vi "Tom Comparison.vi"(8 "Settings":T2={"Name of test"="hammer test--hammer test 03", "Date"=timestamp(3831903982 s since 1904-01-01), "Location"="Home", "Template"="ScratchPad", "Soundcard"="1-2 (QUAD-CAPTURE)", "resolution"=32, "Sampling rate"=48000, "Ch1 Gain "=0.0, "Ch2 Gain"=0.0, "Sample time (s)"=0.3, "Pre-trigger (s)"=0.001, "Hammer Threshold"=0.01, "Positions"=2, "Taps/Position"=5, "Set Names"="H", "Freq resolution"=1.0, "Hammer cutoff"=0.0016020942408376962, "Mic cutoff"=0.06, "Double bounce "=0.01, "Hammer Cal"=1.0, "dB Offset"=0.0, "Accel Cal"=1.0, "Vibrometer Cal"=40.0, "Mic Cal"=66.0, "Output"=0, "Voltage Cal"=1.0, "Vibrometer Port"="ASRL27::INSTR", "Range"=20, "High Pass"=0, "Bandwidth"=25, "X Range"=[{"Minimum"=200.0, "Maximum"=20000.0, "Increment"=10.0, "Minor Increment"=100.0, "Start"=1000.0}, {"Minimum"=0.0, "Maximum"=0.002, "Increment"=0.0005, "Minor Increment"=0.0001, "Start"=0.0}, {"Minimum"=-0.02, "Maximum"=0.3, "Increment"=0.1, "Minor Increment"=0.01, "Start"=0.0}, {"Minimum"=150.0, "Maximum"=10000.0, "Increment"=10.0, "Minor Increment"=100.0, "Start"=1000.0}], "Y Range"=[{"Minimum"=-25.0, "Maximum"=0.0, "Increment"=5.0, "Minor Increment"=1.0, "Start"=-25.0}, {"Minimum"=-0.01, "Maximum"=0.1, "Increment"=0.025, "Minor Increment"=0.005, "Start"=0.0}, {"Minimum"=-1.0, "Maximum"=1.0, "Increment"=0.5, "Minor Increment"=0.1, "Start"=-1.0}, {"Minimum"=0.0, "Maximum"=40.0, "Increment"=2.0, "Minor Increment"=0.5, "Start"=0.0}], "dB Spread"=40.0, "Trigger"=0, "Ch_1"=2, "Ch_2"=1, "flip?"=FALSE, "60Hz"=FALSE, "Time offset"=0.0, "Piezo Cal"=1.0, "Default Notes"="location (e.g., JC workshop, Oberlin acoustics, etc.)\nname of experiment (if applicable) \nnames of researchers\n\nInstrument Information:\ninstrument (e.g., violin, viola, cello, guitar, mandolin, etc.) \nmodel (e.g., Titian Strad, Guadagnini, personal, etc.) \nmaker name\nmaker ID (e.g., serial number)\nyear built (4 digits)\ncountry of origin \nsession (e.g. Oberlin 2017, VSA 2008) \nmaking school (e.g. Old Italian) \n\nMeasurement Information:\ntype (Radiation, admittance, modal analysis, taptones, etc.) \nprotocol (HV24, etc.)\n"} {"Ch_2" min=1 step=1; "Ch_1" min=1 max=100 step=1; "Trigger" items=["Hammer (force)", "Self-tap", "Spacebar"]; "Bandwidth" items=["1 kHz"=1, "5 kHz"=5, "10 kHz"=10, "25 kHz"=25, "50 kHz"=50, "100 kHz"=100]; "High Pass" items=["Off", "13 Hz", "104 Hz"]; "Range" items=["10 mm/s"=1, "20 mm/s"=2, "50 mm/s"=5, "100 mm/s"=10, "200 mm/s"=20, "500 mm/s"=50, "1 m/s"=100, "2 m/s"=200]; "Output" items=["Accelerometer", "Speed (from acceleration)", "Microphone", "Vibrometer", "Piezo"]; "Voltage Cal" format="%#_13g"; "Ch2 Gain" format="%#_13g"; "Ch1 Gain" format="%#_13g"; "Double bounce" min=0.0; "Mic cutoff" min=0.0 format="%#_4g"; "Hammer cutoff" min=0.0 format="%#_4g"; "Freq resolution" min=0.0; "Pre-trigger (s)" format="%#_13g"; "Date" format="%<%H:%M\n%d/%m/%y>T"; "resolution" items=["16 bit"=16, "24 bit"=24, "32 bit"=32]; "Sampling rate" items=["22050 samp/s"=22050, "44100 samp/s"=44100, "48000 samp/s"=48000]}, 11 "Old Files":T3[](array[typedef])) -> ()   [LabVIEW 2022 SP3]
uses:
  Curtin1_Label.ctl
  PreferencesControl.ctl
  GraphType.ctl
panel:
  in  "default":T1={"Name"="Hammer Cutoff 1", "Color"=16777216, "Style"=2, "Point Style"=13, "Name Visible"=FALSE, "Allow Drag"=TRUE, "Cursor Mode"=0, "Plot"=0, "Index"=0, "Position"={"X"=0.0011510989010989011, "Y"=0.0}, "X Scale"=0, "Y Scale"=0, "Watch Plots"=[], "Watch All Plots"=FALSE, "Plot Area"=0, "Label Offset"={"X"=-5.886970172684896e-07, "Y"=0.013114754098360656}}
  out "Hammer Spectra":cluster{dbl, "df":dbl, "FFT {X}":dbl[]}[](graph)=[{1.0, "df"=1.0, "FFT {X}"=array[24000 elements]}]
  out "Microphone Spectra":cluster{"x0":dbl, "df":dbl, dbl[]}[](graph)
  out "Average FRF":cluster{dbl, "df":dbl, dbl[]}[](graph)
  out "Hammer Data":cluster{dbl, "dt":dbl, "Y":dbl[]}[](graph)
  out "Microphone Data":cluster{dbl, "dt":dbl, "Y":dbl[]}[](graph)
  in  "filter":bool
  in  "Data sets":i32[](listbox)
  in  "stop":bool
  # "This looks at the effects of cutoff choice in comparing different hammers.  The filter button simply coerces every value below zero on the hammer reading (a digital diode)"
  # "Tom's Analysis"
  # "Hz"
  # "dB"
  # "dB"
  # "sec"
  # "sec"
  # "mV/Pa"
  # "mV/m/s2"
  # "mV/mm/s"
  # "V/N"
  # "sec"
  # "sec"
  # "mV/N"
  # "a.u."
  # "a.u."
  # "sec"
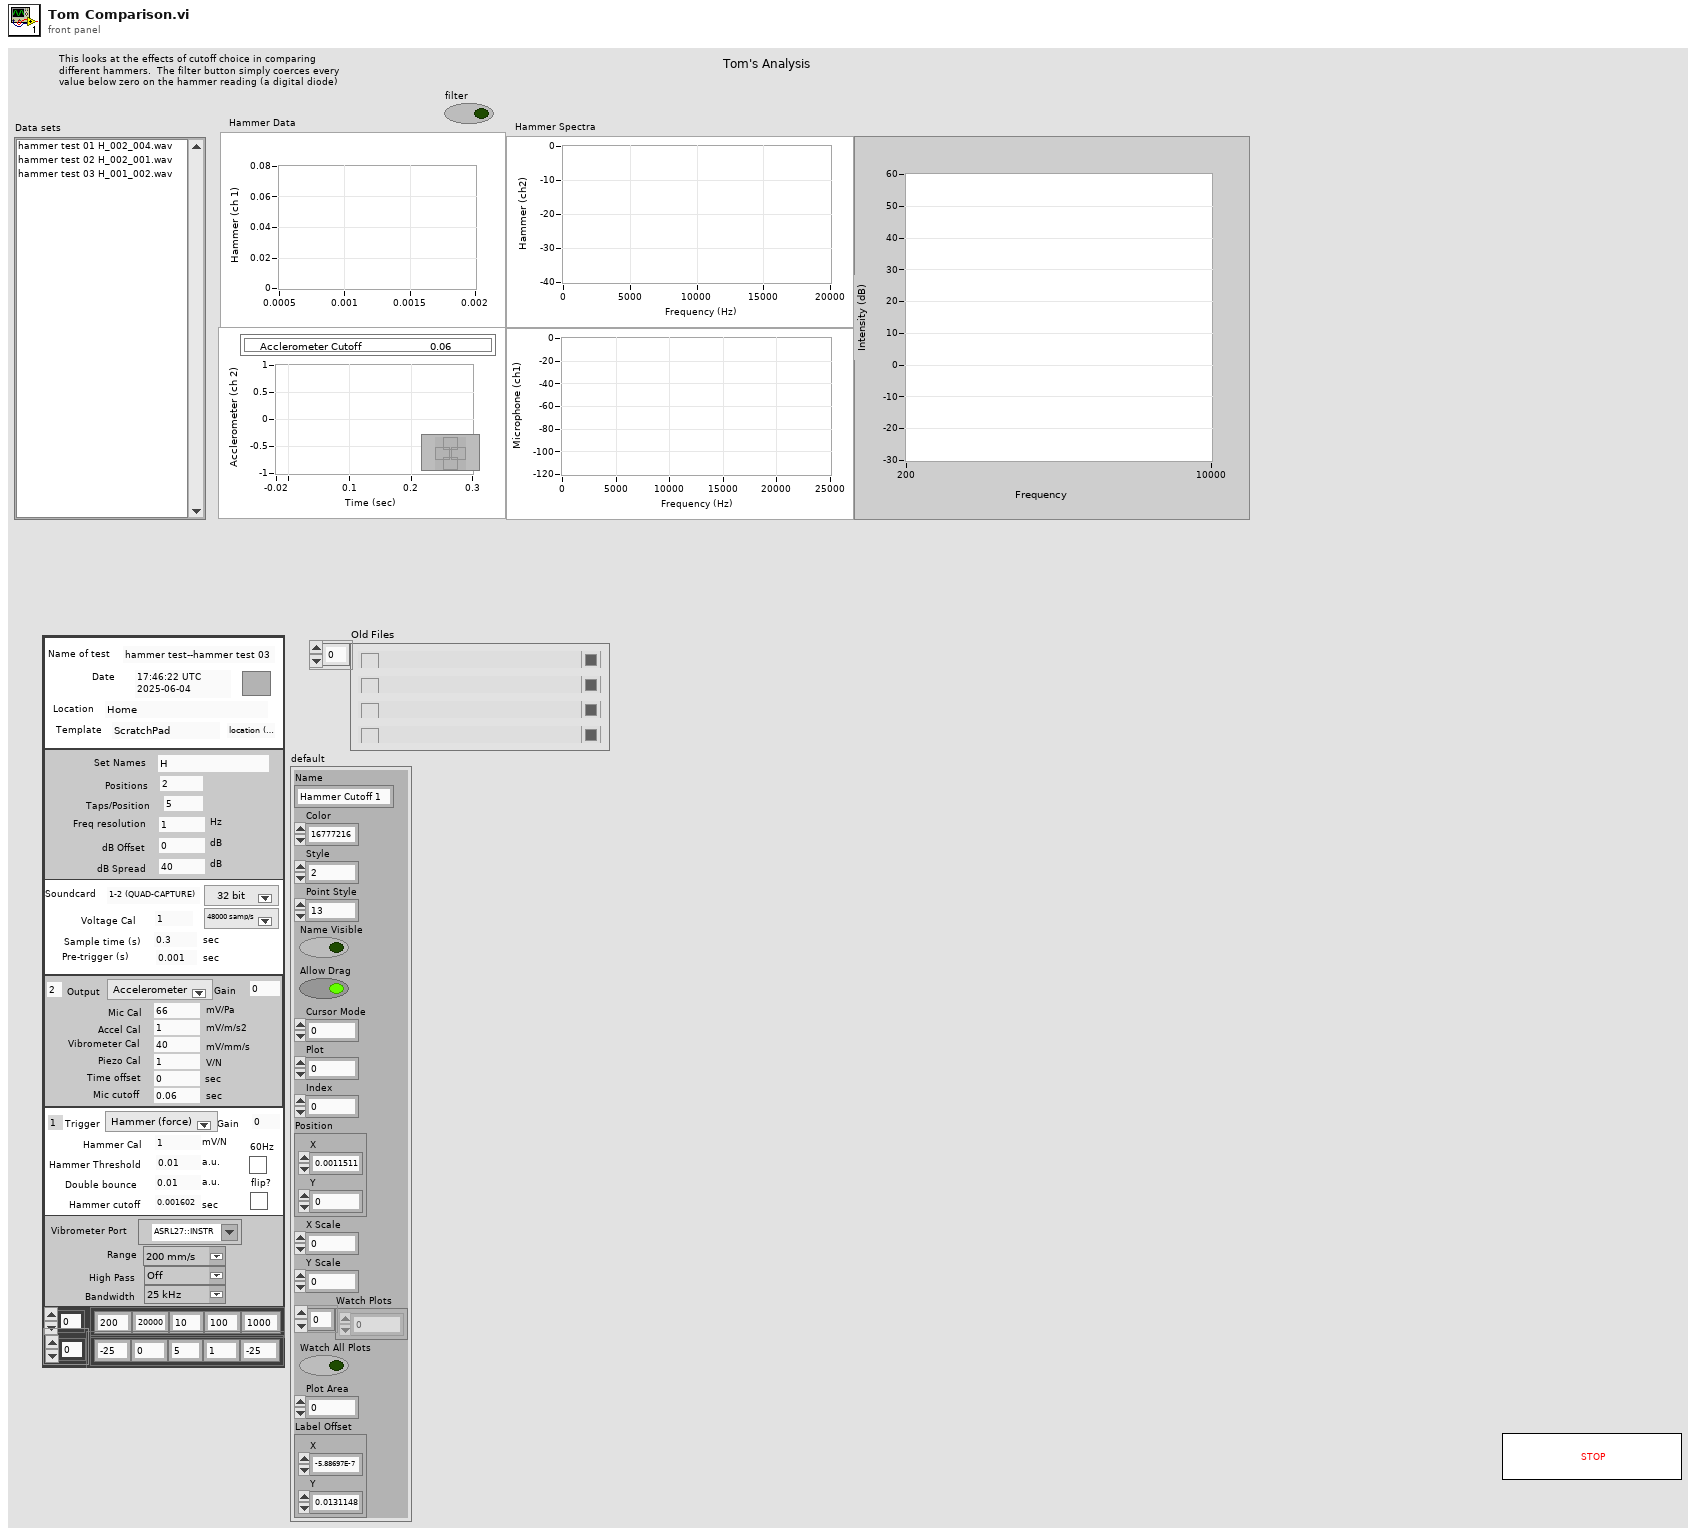
[diagram p1: front panel]
types:
  T1 = cluster{"Name":string, "Color":u32, "Style":u8, "Point Style":u8, "Name Visible":bool, "Allow Drag":bool, "Cursor Mode":u32, "Plot":i32, "Index":i32, "Position":cluster{"X":dbl, "Y":dbl}, "X Scale":u32, "Y Scale":u32, "Watch Plots":i32[], "Watch All Plots":bool, "Plot Area":i32, "Label Offset":cluster{"X":dbl, "Y":dbl}}
  T2 = typedef "PreferencesControl.ctl" = cluster{"Name of test":string, "Date":timestamp, "Location":string, "Template":string, "Soundcard":string, "resolution":u16, "Sampling rate":u16, "Ch1 Gain ":dbl, "Ch2 Gain":dbl, "Sample time (s)":dbl, "Pre-trigger (s)":dbl, "Hammer Threshold":dbl, "Positions":i16, "Taps/Position":i16, "Set Names":string, "Freq resolution":dbl, "Hammer cutoff":dbl, "Mic cutoff":dbl, "Double bounce ":dbl, "Hammer Cal":dbl, "dB Offset":dbl, "Accel Cal":dbl, "Vibrometer Cal":dbl, "Mic Cal":dbl, "Output":u16, "Voltage Cal":dbl, "Vibrometer Port":refnum<visa-resource-name>, "Range":u16, "High Pass":u16, "Bandwidth":u16, "X Range":cluster{"Minimum":dbl, "Maximum":dbl, "Increment":dbl, "Minor Increment":dbl, "Start":dbl}[], "Y Range":cluster{"Minimum":dbl, "Maximum":dbl, "Increment":dbl, "Minor Increment":dbl, "Start":dbl}[], "dB Spread":dbl, "Trigger":u16, "Ch_1":u8, "Ch_2":u8, "flip?":bool, "60Hz":bool, "Time offset":dbl, "Piezo Cal":dbl, "Default Notes":string}
  T3 = typedef "Curtin1_Label.ctl" = cluster{"Show?":bool, "Name":string, "Color":u32, "Path":path, "Show Notes":bool}
  T4 = typedef "GraphType.ctl" = u16
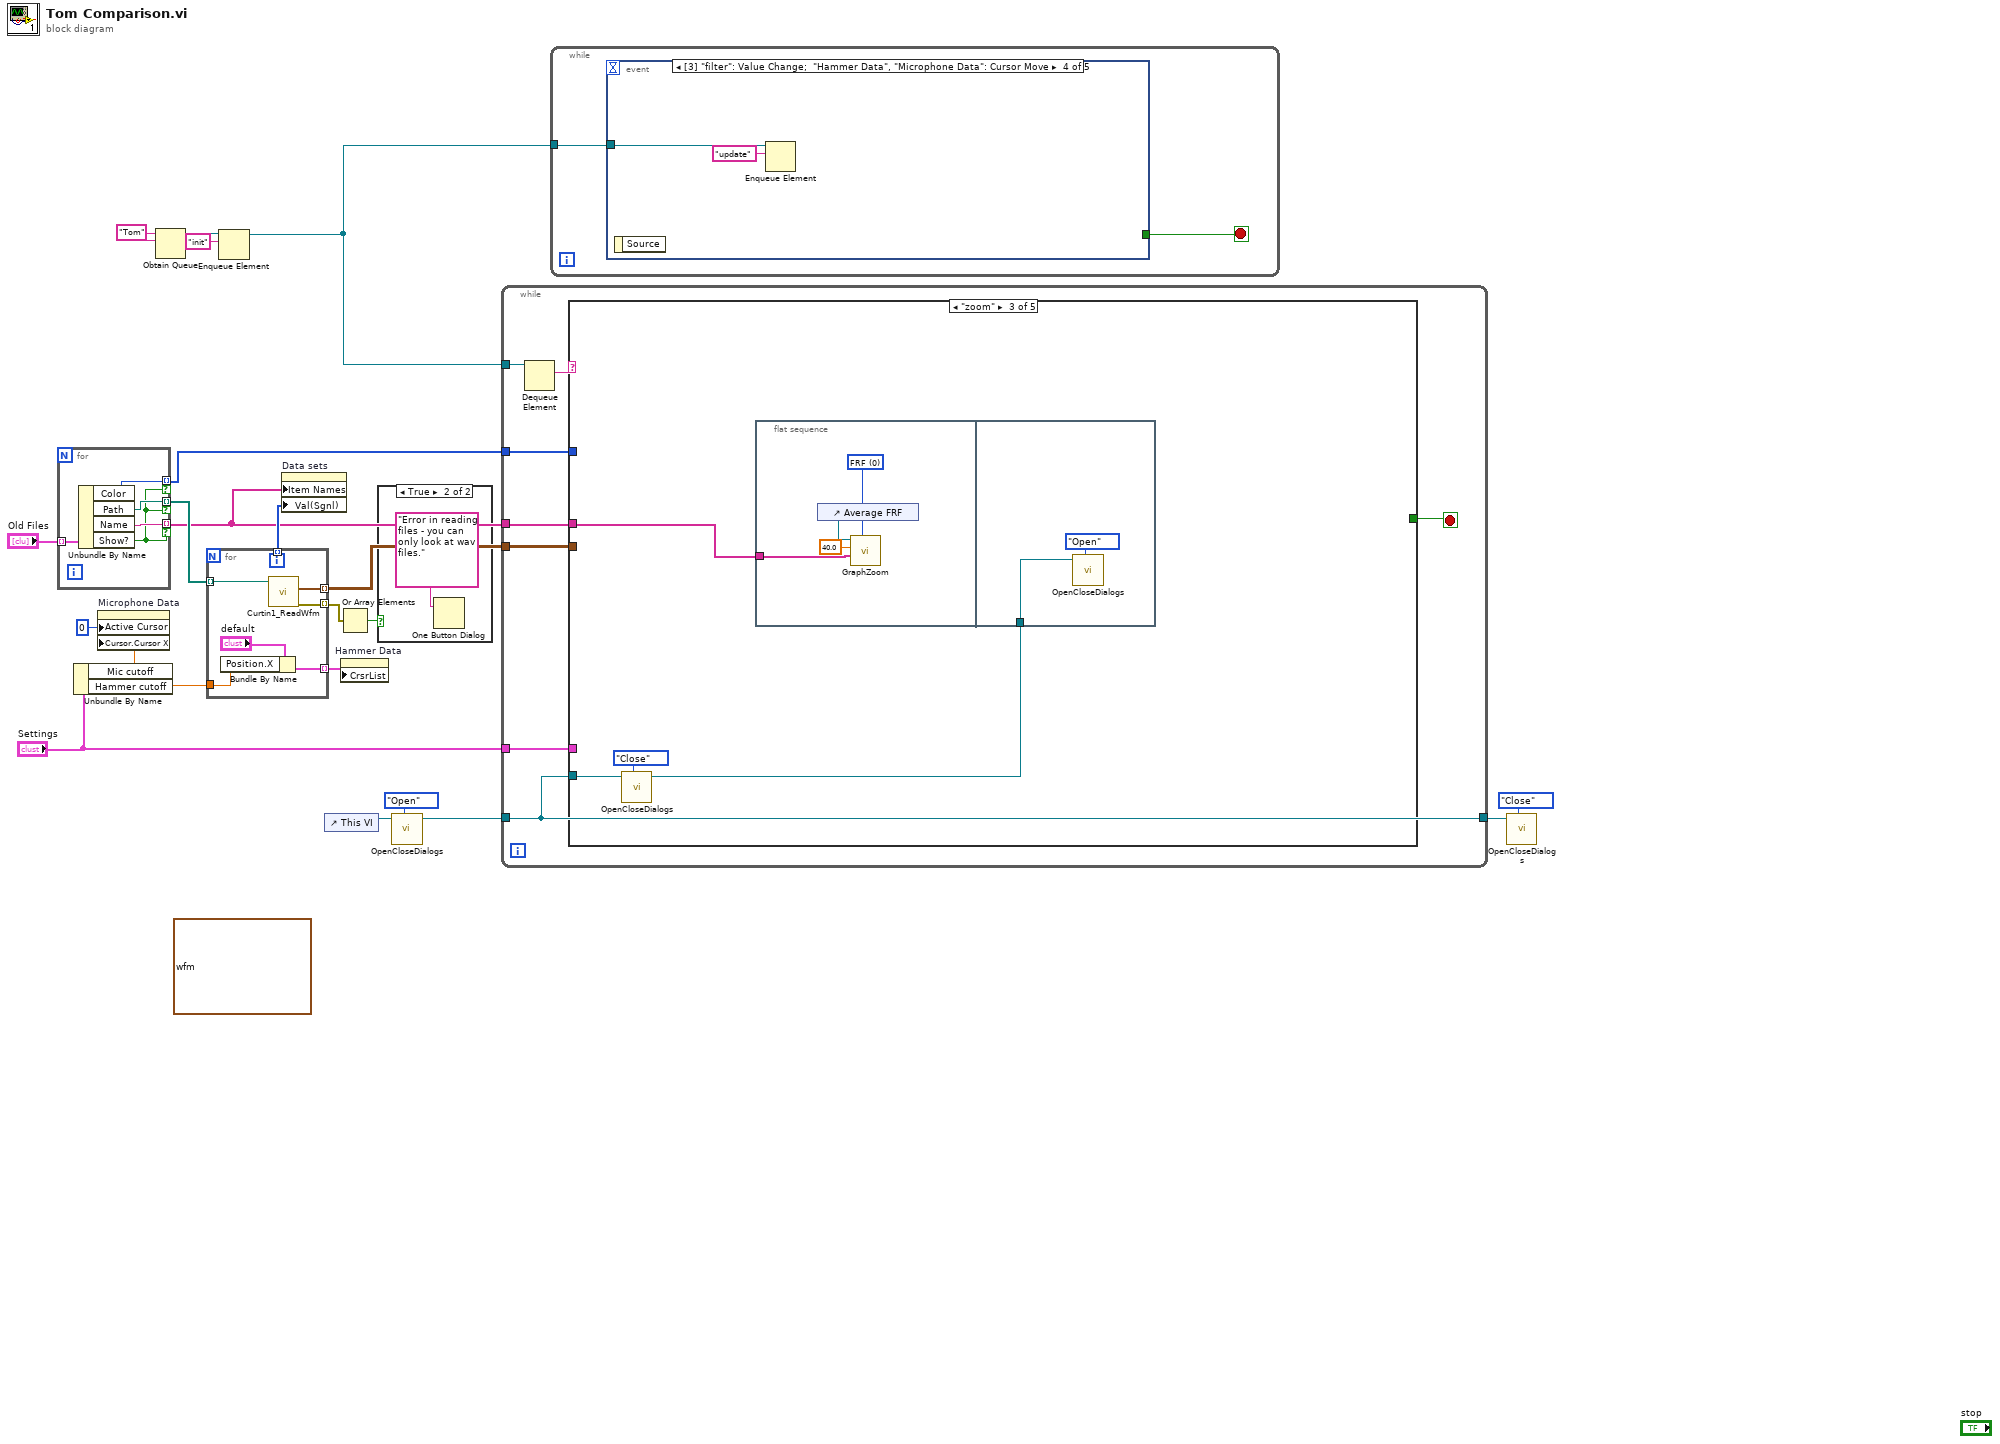
[diagram p0: block diagram]
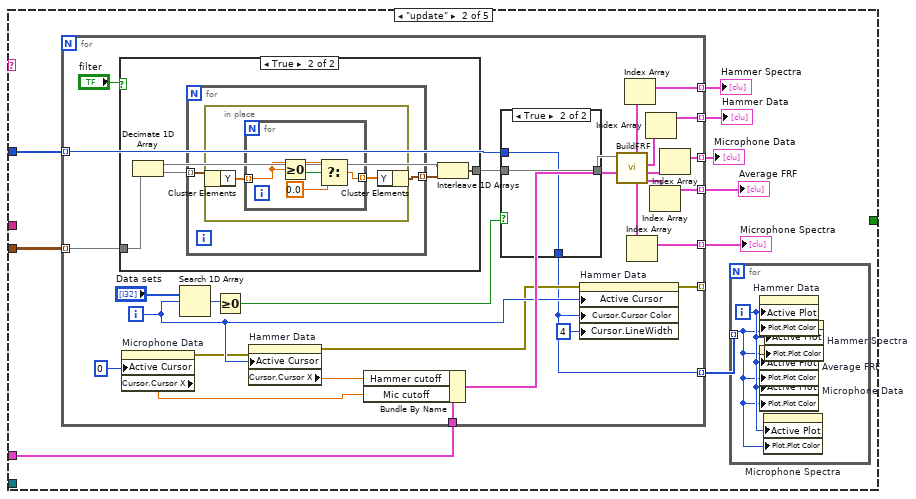
[diagram p4: hidden frame]
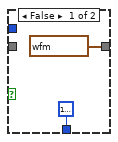
[diagram p5: hidden frame]
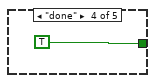
[diagram p7: hidden frame]
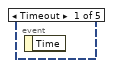
[diagram p9: hidden frame]
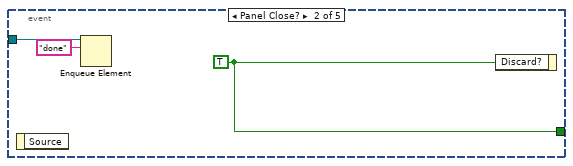
[diagram p10: hidden frame]
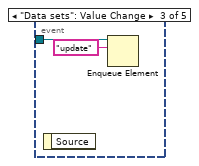
[diagram p11: hidden frame]
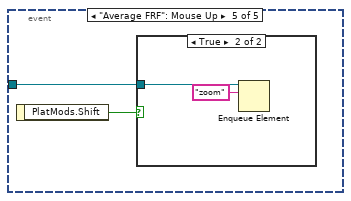
[diagram p12: hidden frame]
diagram:
  w21 = "Tom" ("name (unnamed)")
  (unwired) waveform(dbl)[] [{"t0"=timestamp(0 s since 1904-01-01), "dt"=2.0833333333333333e-05, "Y"=array[14400 elements]}, {"t0"=timestamp(0 s since 1904-01-01), "dt"=2.0833333333333333e-05, "Y"=array[14400 elements]}, {"t0"=timestamp(0 s since 1904-01-01), "dt"=2.0833333333333333e-05, "Y"=array[14400 elements]}, {"t0"=timestamp(0 s since 1904-01-01), "dt"=2.0833333333333333e-05, "Y"=array[14400 elements]}] ("Data In")
  n1 = for {
    tunnel: "Old Files" -> [w27] mode=indexing
    tunnel: [w26] -> w14 mode=indexing if=w23
    tunnel: [w25] -> w17 mode=indexing if=w23
    tunnel: [w24] -> w6 mode=indexing if=w23
    n2 = Unbundle By Name(w27) -> ("Color"=w24:u32, "Path"=w25:path, "Name"=w26:string, "Show?"=w23:bool)
  }
  n3 = Unbundle By Name("Settings") -> ("Mic cutoff"=w9:dbl, "Hammer cutoff"=w11:dbl)
  n4 = property on="Microphone Data" class="WFGraph (strict)"("Active Cursor"=u32 0, "Cursor.Cursor X"=w9) -> ()  [unwired: 2 in, 2 out]
  n5 = Obtain Queue(name (unnamed)=w21, element data type=w21) -> (queue out=w22:refnum<queue>)  [unwired: 3 in, 2 out]
  n6 = for {
    tunnel: w17 -> [w34] mode=indexing
    tunnel: [w33] -> w16 mode=indexing
    tunnel: [w32] -> w15 mode=indexing
    tunnel: [w29] -> w12 mode=indexing
    tunnel: [w31] -> w8 mode=indexing
    tunnel: w11 -> [w28]
    i -> [w32]
    n7 = Bundle By Name(cluster="default", "Position.X"=w28) -> (w29:T1)
    n8 = call "Curtin1_ReadWfm.vi"("appended path"=w34) -> ("error out"=w31:errorcluster, "all waveforms in record"=w33:waveform(dbl)[])  [unwired: 9 in]
  }
  n9 = Enqueue Element(queue=w22, element="init") -> (queue out=w19:refnum<queue>)  [unwired: 2 in, 2 out]
  n10 = property on="Data sets" class="LstBox (strict)"("Item Names"=w14, "Val(Sgnl)"=w15) -> ()  [unwired: 2 in, 2 out]
  n11 = control-ref of="This VI"() -> (w4:refnum<vi>)
  n12 = Or Array Elements(Boolean array=w8) -> (logical OR=w7:bool)
  n13 = property on="Hammer Data" class="WFGraph (strict)"("CrsrList"=w12) -> ()  [unwired: 2 in, 2 out]
  n14 = case shown="True" w7 {
    frame False {
    }
    frame True {
      n15 = One Button Dialog(message="Error in reading files - you can only look at wav files.") -> ()  [unwired: 1 in, 1 out]
    }
  }
  n16 = call "OpenCloseDialogs.vi"("Task"=enum16{"Open", "Close"}."Open", "VI in"=w4) -> ("VI out"=w2:refnum<vi>)  [unwired: 8 in, 1 out]
  n17 = while {
    tunnel: w19 -> [w43]
    tunnel: "Settings" -> [w40]
    tunnel: w16 -> [w39]
    tunnel: w14 -> [w38]
    tunnel: w6 -> [w37]
    tunnel: w2 -> [w36]
    tunnel: [w36] -> w1
    stop <- w41 stop-if-true
    n18 = Dequeue Element(queue=w43) -> (element=w42:string)  [unwired: 2 in, 3 out]
    n19 = case shown="\"zoom\"" w42 {
      tunnel: w39 -> [_ w52 _ _ _]
      tunnel: [_ _ _ TRUE ("Discard?") _] -> w41
      tunnel: w40 -> [_ w46 _ _ _]
      tunnel: w38 -> [_ _ w105 _ _]
      tunnel: w37 -> [_ w45 _ _ _]
      tunnel: w36 -> [_ _ w103 _ _]
      frame Default {
      }
      frame "update" {
        n20 = for {
          tunnel: w52 -> [w83] mode=indexing
          tunnel: [w68] -> w51 mode=indexing
          tunnel: [w70] -> w50 mode=indexing
          tunnel: [w72] -> w49 mode=indexing
          tunnel: [w67] -> w48 mode=indexing
          tunnel: [w73] -> w47 mode=indexing
          tunnel: [w66] -> _ mode=indexing
          tunnel: w46 -> [w63]
          tunnel: w45 -> [w56] mode=indexing
          tunnel: [w55] -> w44 mode=indexing
          i -> [w59]
          n21 = case shown="True" "filter" {
            tunnel: w83 -> [w88 w93]
            tunnel: [w88 w89] -> w78
            frame False {
            }
            frame True {
              n22 = Decimate 1D Array(w93) -> (w90:waveform(dbl)[], w92:waveform(dbl)[])
              n23 = for {
                tunnel: w92 -> [w95] mode=indexing
                tunnel: [w94] -> w91 mode=indexing
                n24 = in-place {
                  n25 = in-place-cluster #1(w95) -> ("Y"=w97:dbl[])
                  n26 = for {
                    tunnel: w97 -> [w99] mode=indexing
                    tunnel: [w98] -> w96 mode=indexing
                    n27 = Greater Or Equal To 0?(x=w99) -> (x >= 0?=w101:bool)
                    n28 = Select(t=w99, s=w101, f=0.0) -> (s? t:f=w98:dbl)
                  }
                  n29 = in-place-cluster #1("Y"=w96) -> (w94:waveform(dbl))
                }
              }
              n30 = Interleave 1D Arrays(w90, w91) -> (w89:waveform(dbl)[])
            }
          }
          n31 = property on="Microphone Data" class="WFGraph (strict)"("Active Cursor"=u32 0) -> (error out=w58:errorcluster, "Cursor.Cursor X"=w60:dbl)  [unwired: 2 in, 1 out]
          n32 = Search 1D Array(1D array="Data sets", element=w59) -> (index of element=w80:i32)  [unwired: 1 in]
          n33 = Greater Or Equal To 0?(x=w80) -> (x >= 0?=w79:bool)
          n34 = property on="Hammer Data" class="WFGraph (strict)"(error in=w58, "Active Cursor"=w59) -> (error out=w57:errorcluster, "Cursor.Cursor X"=w64:dbl)  [unwired: 1 in, 1 out]
          n35 = Bundle By Name(cluster=w63, "Hammer cutoff"=w64, "Mic cutoff"=w60) -> (w62:T2)
          n36 = case shown="True" w79 {
            tunnel: [waveform(dbl)[] [{"t0"=timestamp(0 s since 1904-01-01), "dt"=1.0, "Y"=[1.0]}, {"t0"=timestamp(0 s since 1904-01-01), "dt"=1.0, "Y"=[]}] ("all waveforms in record") w87] -> w74
            tunnel: w78 -> [_ w87]
            tunnel: w56 -> [_ w86]
            tunnel: [u32 16777216 ("Cursor.Cursor Color") w86] -> w55
            frame False {
            }
            frame True {
            }
          }
          n37 = property on="Hammer Data" class="WFGraph (strict)"(error in=w57, "Active Cursor"=w59, "Cursor.Cursor Color"=w55, "Cursor.LineWidth"=u8 4 ("Cursor.Line Width")) -> (error out=w66:errorcluster)  [unwired: 1 in, 1 out]
          n38 = call "BuildFRF.vi"("Settings"=w62, "Data In"=w74) -> ("Average FRF"=w77:cluster{dbl, "df":dbl, dbl[]}[], "Microphone"=w69:cluster{dbl, "dt":dbl, "Y":dbl[]}[], "Hammer"=w71:cluster{dbl, "dt":dbl, "Y":dbl[]}[], "Microphone Spectra"=w76:cluster{"x0":dbl, "df":dbl, dbl[]}[], "Hammer Spectra"=w75:cluster{dbl, "df":dbl, "FFT {X}":dbl[]}[])  [unwired: 4 in, 1 out]
          n39 = Index Array(array=w75) -> (element=w73:cluster{dbl, "df":dbl, "FFT {X}":dbl[]})  [unwired: 1 in]
          n40 = Index Array(array=w76) -> (element=w67:cluster{"x0":dbl, "df":dbl, dbl[]})  [unwired: 1 in]
          n41 = Index Array(array=w71) -> (element=w72:cluster{dbl, "dt":dbl, "Y":dbl[]})  [unwired: 1 in]
          n42 = Index Array(array=w77) -> (element=w68:cluster{dbl, "df":dbl, dbl[]})  [unwired: 1 in]
          n43 = Index Array(array=w69) -> (element=w70:cluster{dbl, "dt":dbl, "Y":dbl[]})  [unwired: 1 in]
        }
        "Microphone Data" <- w50
        "Hammer Data" <- w49
        "Hammer Spectra" <- w47
        "Microphone Spectra" <- w48
        "Average FRF" <- w51
        n44 = for {
          tunnel: w44 -> [w53] mode=indexing
          i -> [w54]
          n45 = property on="Hammer Data" class="WFGraph (strict)"("Active Plot"=w54, "Plot.Plot Color"=w53) -> ()  [unwired: 2 in, 2 out]
          n46 = property on="Average FRF" class="WFGraph (strict)"("Active Plot"=w54, "Plot.Plot Color"=w53) -> ()  [unwired: 2 in, 2 out]
          n47 = property on="Microphone Data" class="WFGraph (strict)"("Active Plot"=w54, "Plot.Plot Color"=w53) -> ()  [unwired: 2 in, 2 out]
          n48 = property on="Microphone Spectra" class="WFGraph (strict)"("Active Plot"=w54, "Plot.Plot Color"=w53) -> ()  [unwired: 2 in, 2 out]
          n49 = property on="Hammer Spectra" class="WFGraph (strict)"("Active Plot"=w54, "Plot.Plot Color"=w53) -> ()  [unwired: 2 in, 2 out]
        }
      }
      frame "zoom" {
        n50 = call "OpenCloseDialogs.vi"("Task"=enum16{"Open", "Close"}."Close", "VI in"=w103) -> ("VI out"=w102:refnum<vi>)  [unwired: 8 in, 1 out]
        n51 = flat-sequence {
          tunnel: w105 -> [w106]
          tunnel: w102 -> [w110]
          frame #0 {
            w107 = T4 0 items=["FRF", "rad phase unwrapped", "deg phase unwrapped", "rad phase wrapped", "deg phase wrapped", "White Plots", "MJ Map", "Real and Imaginary"] ("Plot")
            n52 = control-ref of="Average FRF"() -> (w108:refnum<vi>)
            n53 = call "GraphZoom.vi"("Plot"=w107, "Names"=w106, "dB Range"=40.0, "Graph"=w108) -> ()  [unwired: 8 in]
          }
          frame #1 {
            n54 = call "OpenCloseDialogs.vi"("Task"=enum16{"Open", "Close"}."Open", "VI in"=w110) -> ()  [unwired: 8 in, 2 out]
          }
        }
      }
      frame "done" {
      }
      frame "init" {
      }
    }
  }
  n55 = while {
    tunnel: w19 -> [w113]
    stop <- w114 stop-if-true
    n56 = event shown="[3] \"filter\": Value Change;  \"Hammer Data\", \"Microphone Data\": Cursor Move" {
      selector: _ -> [_ _ _ _ _]
      dyn-events: _ -> [_ _ _ _ _]
      timeout: _ -> [_ _ _ _ _]
      tunnel: [_ w117 _ _ _] -> w114
      tunnel: w113 -> [_ w115 w118 w120 w123]
      event Timeout {
        n57 = event-data() -> ()  [unwired: 1 in, 1 out]
      }
      event Panel Close? {
        w117 = TRUE ("Discard?")
        n58 = event-data() -> ()  [unwired: 1 in, 1 out]
        n59 = Enqueue Element(queue=w115, element="done") -> ()  [unwired: 2 in, 3 out]
        n60 = event-data("Discard?"=w117) -> ()  [unwired: 1 in, 1 out]
      }
      event "Data sets": Value Change {
        n61 = event-data() -> ()  [unwired: 1 in, 1 out]
        n62 = Enqueue Element(queue=w118, element="update") -> ()  [unwired: 2 in, 3 out]
      }
      event "filter": Value Change; "Hammer Data", "Microphone Data": Cursor Move {
        n63 = event-data() -> ()  [unwired: 1 in, 1 out]
        n64 = Enqueue Element(queue=w120, element="update") -> ()  [unwired: 2 in, 3 out]
      }
      event "Average FRF": Mouse Up {
        n65 = event-data() -> ("PlatMods.Shift"=w122:bool)  [unwired: 1 in]
        n66 = case shown="True" w122 {
          tunnel: w123 -> [_ w124]
          frame False {
          }
          frame True {
            n67 = Enqueue Element(queue=w124, element="zoom") -> ()  [unwired: 2 in, 3 out]
          }
        }
      }
    }
  }
  n68 = call "OpenCloseDialogs.vi"("Task"=enum16{"Open", "Close"}."Close", "VI in"=w1) -> ()  [unwired: 8 in, 2 out]
